vi "285_Move.vi"(7 "VISA resource name out":refnum<visa-resource-name>, 8 "error in (no error)":errorcluster caption="错误输入（无错误）", 9 "Abso_Z":dbl, 10 "Abso_Y":dbl, 11 "Abso_X":dbl) -> (0 "error out":errorcluster caption="错误输出", 1 "read buffer 2":string, 2 "read buffer":string, 3 "VISA resource name out 2":refnum<visa-resource-name>)   [LabVIEW 2018]
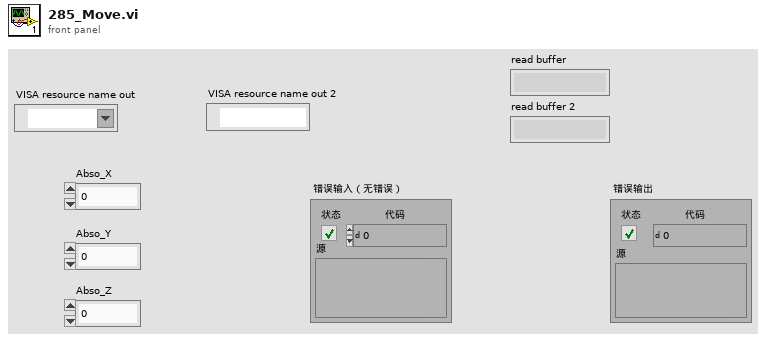
[diagram p1: front panel]
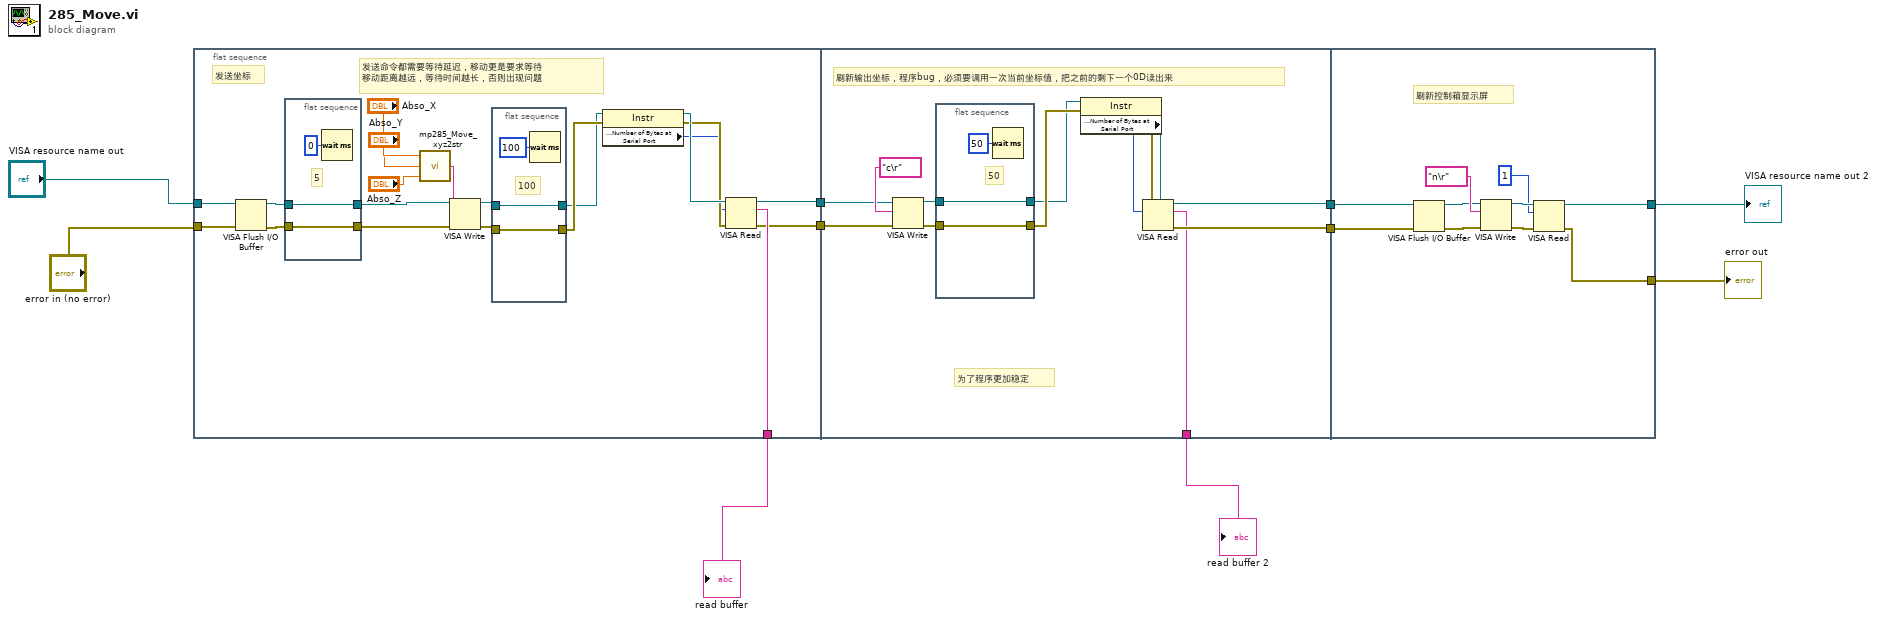
[diagram p0: block diagram]
diagram:
  n1 = flat-sequence {
    tunnel: "error in (no error)" -> [w24]
    tunnel: "VISA resource name out" -> [w25]
    tunnel: [w26] -> w8
    tunnel: [w18] -> w7
    tunnel: [w19] -> w6
    tunnel: w7 -> [w41]
    tunnel: w6 -> [w40]
    tunnel: [w39] -> w5
    tunnel: [w38] -> w4
    tunnel: [w37] -> w3
    tunnel: w5 -> [w58]
    tunnel: w4 -> [w57]
    tunnel: [w54] -> w2
    tunnel: [w53] -> w1
    frame #0 {
      # "发送命令都需要等待延迟，移动更是要求等待\n移动距离越远，等待时间越长，否则出现问题"
      # "发送坐标"
      n2 = VISA Flush I/O Buffer(VISA resource name=w25, error in (no error)=w24) -> (VISA resource name out=w23:refnum<visa-resource-name>, error out=w22:errorcluster)  [unwired: 1 in]
      n3 = flat-sequence {
        tunnel: [w35] -> w21
        tunnel: w23 -> [w35]
        tunnel: [w34] -> w20
        tunnel: w22 -> [w34]
        frame #0 {
          # "5"
          n4 = Wait (ms)(milliseconds to wait=u32 0 ("等待时间（毫秒）")) -> ()  [unwired: 1 out]
        }
      }
      n5 = call "mp285_Move_xyz2str.vi"("Z轴"="Abso_Z", "Y轴"="Abso_Y", "X轴"="Abso_X") -> ("发送至串口的字符串"=w30:string)
      n6 = VISA Write ("VISA写入")(VISA resource name=w21, write buffer=w30, error in (no error)=w20) -> (VISA resource name out=w14:refnum<visa-resource-name>, error out=w13:errorcluster)  [unwired: 1 out]
      n7 = flat-sequence {
        tunnel: w14 -> [w32]
        tunnel: w13 -> [w31]
        tunnel: [w32] -> w11
        tunnel: [w31] -> w12
        frame #0 {
          # "100"
          n8 = Wait (ms)(milliseconds to wait=u32 100 ("等待时间（毫秒）")) -> ()  [unwired: 1 out]
        }
      }
      n9 = property class="Instr"(reference=w11, error in=w12) -> (reference out=w17:refnum<visa-resource-name>, error out=w16:errorcluster, "Serial Settings:Number of Bytes at Serial Port"=w15:u32)
      n10 = VISA Read(VISA resource name=w17, byte count=w15, error in (no error)=w16) -> (VISA resource name out=w18:refnum<visa-resource-name>, read buffer=w26:string, error out=w19:errorcluster)  [unwired: 1 out]
    }
    frame #1 {
      # "为了程序更加稳定"
      # "刷新输出坐标，程序bug，必须要调用一次当前坐标值，把之前的剩下一个0D读出来"
      n11 = VISA Write ("VISA写入")(VISA resource name=w41, write buffer="c\r" ("写入缓冲区"), error in (no error)=w40) -> (VISA resource name out=w46:refnum<visa-resource-name>, error out=w47:errorcluster)  [unwired: 1 out]
      n12 = flat-sequence {
        tunnel: w46 -> [w51]
        tunnel: w47 -> [w50]
        tunnel: [w51] -> w48
        tunnel: [w50] -> w49
        frame #0 {
          # "50"
          n13 = Wait (ms)(milliseconds to wait=u32 50 ("等待时间（毫秒）")) -> ()  [unwired: 1 out]
        }
      }
      n14 = property class="Instr"(reference=w48, error in=w49) -> (reference out=w43:refnum<visa-resource-name>, error out=w42:errorcluster, "Serial Settings:Number of Bytes at Serial Port"=w44:u32)
      n15 = VISA Read(VISA resource name=w43, byte count=w44, error in (no error)=w42) -> (VISA resource name out=w39:refnum<visa-resource-name>, read buffer=w37:string, error out=w38:errorcluster)  [unwired: 1 out]
    }
    frame #2 {
      # "刷新控制箱显示屏"
      n16 = VISA Flush I/O Buffer(VISA resource name=w58, error in (no error)=w57) -> (VISA resource name out=w56:refnum<visa-resource-name>, error out=w55:errorcluster)  [unwired: 1 in]
      n17 = VISA Write ("VISA写入")(VISA resource name=w56, write buffer="n\r" ("写入缓冲区"), error in (no error)=w55) -> (VISA resource name out=w60:refnum<visa-resource-name>, error out=w61:errorcluster)  [unwired: 1 out]
      n18 = VISA Read(VISA resource name=w60, byte count=u32 1 ("字节总数"), error in (no error)=w61) -> (VISA resource name out=w54:refnum<visa-resource-name>, error out=w53:errorcluster)  [unwired: 2 out]
    }
  }
  "error out" <- w1
  "VISA resource name out 2" <- w2
  "read buffer" <- w8
  "read buffer 2" <- w3
